vi "FIRSTSUBVI.vi"(1 "Numeric 2":dbl, 2 "Numeric":dbl) -> (0 "(A+B)/2":dbl)   [LabVIEW 2019]
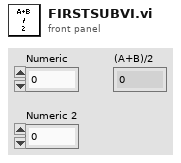
[diagram p1: front panel]
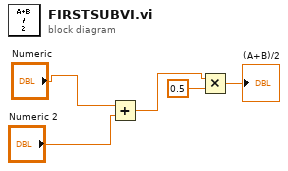
[diagram p0: block diagram]
diagram:
  n1 = Add(x="Numeric", y="Numeric 2") -> (x+y=w3:dbl)
  n2 = Multiply(x=w3, y=0.5) -> (x*y=→"(A+B)/2":dbl)
